vi "LEBITVacuum.ParseAMArray.vi"(3 "AMArray":string[][](array[string])) -> (15 "MKS Measurement":string[](array[string]), 16 "MKS Address Array":i32[][](array[numeric]), 17 "MKS MeasurementServiceID":i32[](array[numeric]), 18 "CRYO Measurement":string[][](array[string]), 19 "CRYO MeasurementServiceID":i32[](array[numeric]))   [LabVIEW 2014, in "LEBITVacuum.lvlib"]
uses:
  LEBITVacuum.lvlib
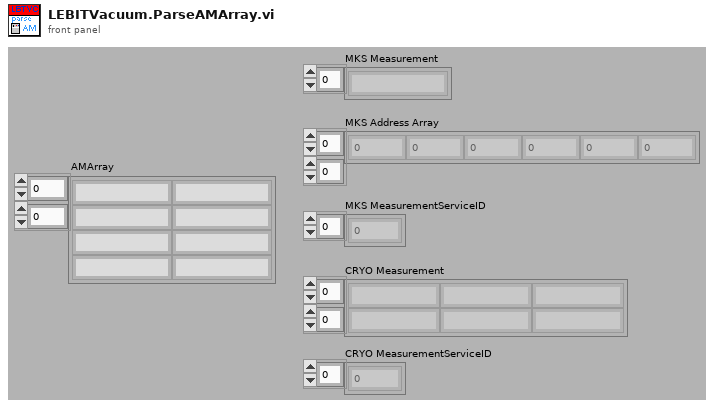
[diagram p1: front panel]
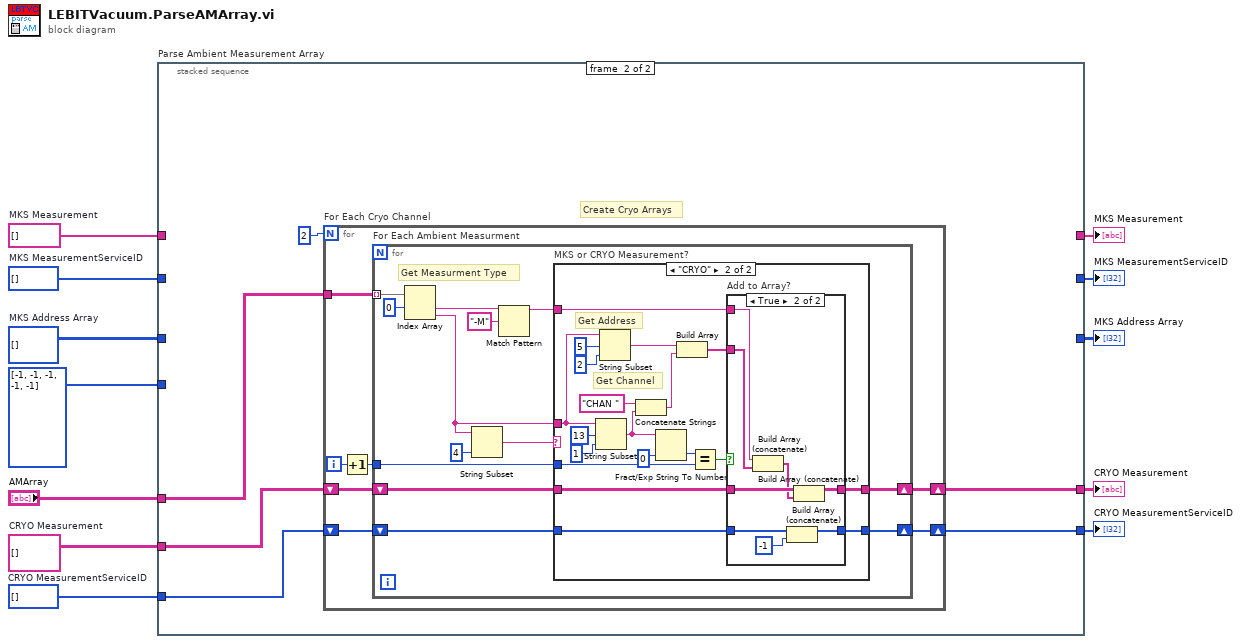
[diagram p0: block diagram]
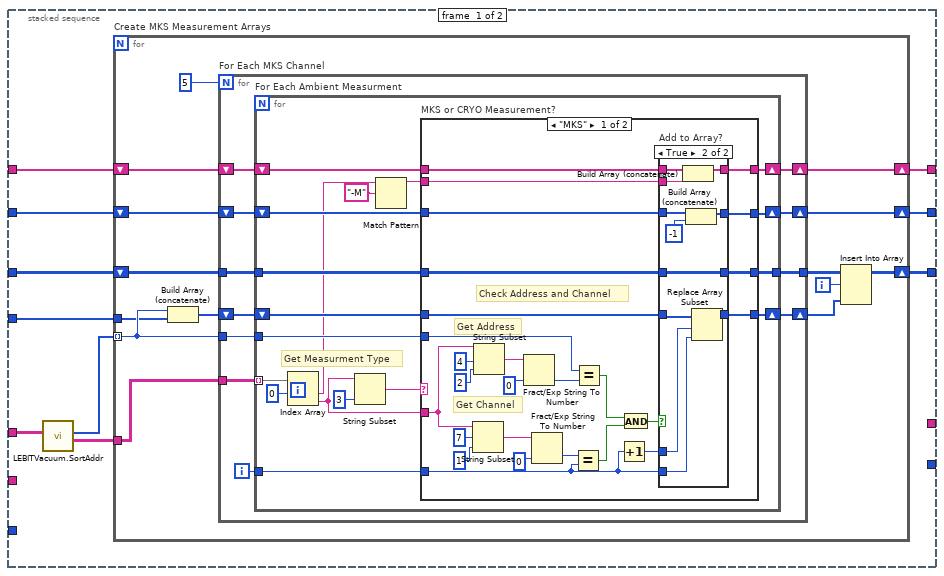
[diagram p2: hidden frame]
diagram:
  w1 = i32[] []  # CRYO MeasurementServiceID
  w2 = string[][] []  # CRYO Measurement
  w6 = i32[] []  # MKS MeasurementServiceID
  w8 = string[] []  # MKS Measurement
  w11 = i32[][] []  # MKS Address Array
  n1 = stacked-sequence "Parse Ambient Measurement Array" {
    tunnel: "AMArray" -> [w22 w115]
    tunnel: w11 -> [w20 _]
    tunnel: [w19 _] -> w10
    tunnel: i32[] [-1, -1, -1, -1, -1] -> [w18 _]
    tunnel: w8 -> [w17 _]
    tunnel: [w16 _] -> w7
    tunnel: w6 -> [w15 _]
    tunnel: [w14 _] -> w5
    tunnel: [_ w114] -> w3
    tunnel: [_ w113] -> w4
    tunnel: w2 -> [_ w112]
    tunnel: w1 -> [_ w111]
    frame #0 {
      n2 = call "LEBITVacuum.SortAddr.vi"("AMArray in"=w22) -> ("AMArray out"=w13:string[][], "MKS Address Array"=w21:i32[])  [unwired: 5 in]
      n3 = for "Create MKS Measurement Arrays" {
        tunnel: w13 -> [w23]
        tunnel: w21 -> [w30] mode=indexing
        shift-right: [w33] -> w19
        shift-left: w20 -> [w32]
        tunnel: w18 -> [w29]
        shift-right: [w25] -> w16
        shift-left: w17 -> [w27]
        shift-right: [w26] -> w14
        shift-left: w15 -> [w24]
        i -> [w34]
        n4 = Build Array (concatenate)(w30, w29) -> (w31:i32[])
        n5 = for "For Each MKS Channel" {
          N: 5 -> [_]
          tunnel: w23 -> [w41]
          tunnel: w30 -> [w47]
          tunnel: w32 -> [w45]
          shift-right: [w42] -> w28
          shift-left: w31 -> [w44]
          tunnel: [w43] -> w35
          shift-right: [w39] -> w25
          shift-left: w27 -> [w40]
          shift-right: [w37] -> w26
          shift-left: w24 -> [w38]
          i -> [w46]
          n6 = for "For Each Ambient Measurment" {
            tunnel: w41 -> [w65] mode=indexing
            tunnel: w47 -> [w63]
            tunnel: w46 -> [w59]
            tunnel: w45 -> [w58]
            tunnel: [w56] -> w43
            shift-right: [w55] -> w42
            shift-left: w44 -> [w57]
            shift-right: [w52] -> w39
            shift-left: w40 -> [w54]
            shift-right: [w51] -> w37
            shift-left: w38 -> [w53]
            # "Get Measurment Type"
            n7 = Index Array(array=w65, index #1=0 ("index")) -> (element #1=w49:string, element #2=w60:string)  [unwired: 1 in]
            n8 = String Subset(string=w60, length (rest)=3 ("length (rest)")) -> (substring=w61:string)  [unwired: 1 in]
            n9 = Match Pattern(string=w49, regular expression="-M") -> (before substring=w48:string)  [unwired: 1 in, 3 out]
            n10 = case "MKS or CRYO Measurement?" shown="\"MKS\"" w61 {
              tunnel: w63 -> [w83 _]
              tunnel: w60 -> [w85 _]
              tunnel: w59 -> [w67 _]
              tunnel: w58 -> [w76 w109]
              tunnel: w57 -> [w80 w110]
              tunnel: [w79 w110] -> w55
              tunnel: [w75 w109] -> w56
              tunnel: w54 -> [w74 w108]
              tunnel: w48 -> [w73 _]
              tunnel: [w72 w108] -> w52
              tunnel: w53 -> [w71 w107]
              tunnel: [w70 w107] -> w51
              frame "MKS" {
                # "Check Address and Channel"
                # "Get Channel"
                # "Get Address"
                n11 = String Subset(string=w85, offset (0)=7, length (rest)=1 ("length (rest)")) -> (substring=w86:string)
                n12 = String Subset(string=w85, offset (0)=4, length (rest)=2 ("length (rest)")) -> (substring=w89:string)
                n13 = Fract/Exp String To Number(string=w89, default (0 dbl)=0 ("length (rest)")) -> (number=w84:i32)  [unwired: 2 in, 1 out]
                n14 = Fract/Exp String To Number(string=w86, default (0 dbl)=0 ("length (rest)")) -> (number=w68:i32)  [unwired: 2 in, 1 out]
                n15 = Equal?(x=w68, y=w67) -> (x = y?=w82:bool)
                n16 = Equal?(x=w83, y=w84) -> (x = y?=w81:bool)
                n17 = Increment(x=w67) -> (x+1=w77:i32)
                n18 = And(x=w81, y=w82) -> (x .and. y?=w78:bool)
                n19 = case "Add to Array?" shown="True" w78 {
                  tunnel: w80 -> [w95 w106]
                  tunnel: w67 -> [_ w104]
                  tunnel: [w95 w105] -> w79
                  tunnel: w77 -> [_ w97]
                  tunnel: w76 -> [w94 w103]
                  tunnel: [w94 w103] -> w75
                  tunnel: w74 -> [w93 w101]
                  tunnel: w73 -> [_ w100]
                  tunnel: [w93 w102] -> w72
                  tunnel: w71 -> [w92 w98]
                  tunnel: [w92 w99] -> w70
                  frame False {
                  }
                  frame True {
                    n20 = Build Array (concatenate)(w101, w100) -> (w102:string[])
                    n21 = Build Array (concatenate)(w98, -1 ("index (row)")) -> (w99:i32[])
                    n22 = Replace Array Subset(array=w106, new element=w104, index=w97) -> (w105:i32[])
                  }
                }
              }
              frame "CRYO", Default {
              }
            }
          }
        }
        n23 = Insert Into Array(array=w35, index (row)=w34, new element=w28) -> (w33:i32[][])  [unwired: 1 in]
      }
    }
    frame #1 {
      # "Create Cryo Arrays"
      n24 = for "For Each Cryo Channel" {
        N: 2 -> [_]
        shift-right: [w121] -> w114
        shift-left: w112 -> [w123]
        shift-right: [w120] -> w113
        shift-left: w111 -> [w122]
        tunnel: w115 -> [w117]
        i -> [w119]
        n25 = Increment(x=w119) -> (x+1=w118:i32)
        n26 = for "For Each Ambient Measurment" {
          tunnel: w118 -> [w133]
          shift-right: [w130] -> w121
          shift-left: w123 -> [w132]
          shift-right: [w129] -> w120
          shift-left: w122 -> [w131]
          tunnel: w117 -> [w128] mode=indexing
          # "Get Measurment Type"
          n27 = Index Array(array=w128, index #1=0 ("index")) -> (element #1=w126:string, element #2=w127:string)  [unwired: 1 in]
          n28 = String Subset(string=w127, length (rest)=4 ("length (rest)")) -> (substring=w134:string)  [unwired: 1 in]
          n29 = Match Pattern(string=w126, regular expression="-M") -> (before substring=w124:string)  [unwired: 1 in, 3 out]
          n30 = case "MKS or CRYO Measurement?" shown="\"CRYO\"" w134 {
            tunnel: w133 -> [_ w153]
            tunnel: w132 -> [w138 w151]
            tunnel: w131 -> [w137 w150]
            tunnel: [w138 w149] -> w130
            tunnel: [w137 w148] -> w129
            tunnel: w124 -> [_ w147]
            tunnel: w127 -> [_ w142]
            frame Default {
            }
            frame "CRYO" {
              # "Get Address"
              # "Get Channel"
              n31 = String Subset(string=w142, offset (0)=13, length (rest)=1 ("length (rest)")) -> (substring=w145:string)
              n32 = String Subset(string=w142, offset (0)=5, length (rest)=2 ("length (rest)")) -> (substring=w141:string)
              n33 = Concatenate Strings("CHAN " ("string"), w145) -> (w139:string)
              n34 = Fract/Exp String To Number(string=w145, default (0 dbl)=0 ("length (rest)")) -> (number=w154:i32)  [unwired: 2 in, 1 out]
              n35 = Build Array(w141, w139) -> (w140:string[])
              n36 = Equal?(x=w154, y=w153) -> (x = y?=w152:bool)
              n37 = case "Add to Array?" shown="True" w152 {
                tunnel: w151 -> [w159 w164]
                tunnel: w150 -> [w158 w166]
                tunnel: [w159 w163] -> w149
                tunnel: [w158 w167] -> w148
                tunnel: w147 -> [_ w160]
                tunnel: w140 -> [_ w161]
                frame False {
                }
                frame True {
                  n38 = Build Array (concatenate)(w160, w161) -> (w162:string[])
                  n39 = Build Array (concatenate)(w166, -1 ("index (row)")) -> (w167:i32[])
                  n40 = Build Array (concatenate)(w164, w162) -> (w163:string[][])
                }
              }
            }
          }
        }
      }
    }
  }
  "MKS Address Array" <- w10
  "MKS Measurement" <- w7
  "MKS MeasurementServiceID" <- w5
  "CRYO MeasurementServiceID" <- w4
  "CRYO Measurement" <- w3
